vi "PWM In (subVI).vi"(0 "PWM Input":bool) -> (1 "Low Period":u32, 2 "High Period":u32)   [LabVIEW 2015]
doc: "This subVI supports a simple PWM measurement. An input signal is measured for its low period and high period."
panel:
  # "This subVI supports a simple PWM measurement.  An input signal is measured for its low period and high period."
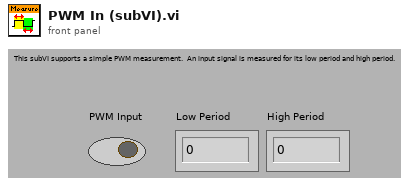
[diagram p1: front panel]
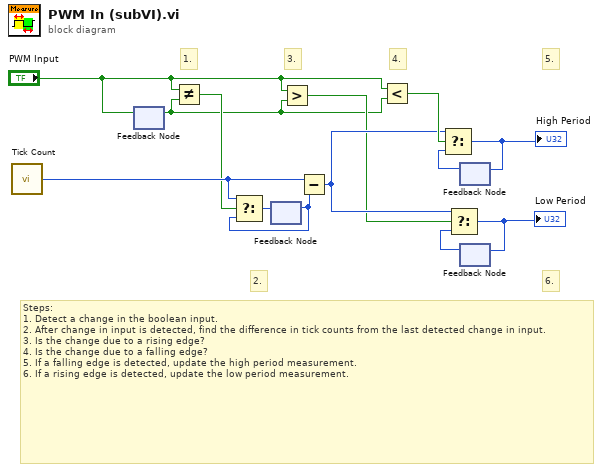
[diagram p0: block diagram]
diagram:
  # "Steps:\n1. Detect a change in the boolean input.\n2. After change in input is detected, find the difference in tick counts from the last detected change in input.\n3. Is the change due to a rising edge?\n4. Is the change due to a falling edge?\n5. If a falling edge is detected, update the high period measurement.\n6. If a rising edge is detected, update the low period measurement."
  # "5."
  # "6."
  # "2."
  # "4."
  # "3."
  # "1."
  n1 = call "Tick Count"() -> ("Tick Count(mSec)"=w13:u32)
  n2 = feedback-in #1("PWM Input") -> ()
  n3 = feedback #1() -> (w8:bool)  [unwired: 1 out]
  n4 = Not Equal?(x="PWM Input", y=w8) -> (x != y?=w9:bool)
  n5 = feedback #2() -> (w2:u32)  [unwired: 1 out]
  n6 = Select(t=w13, s=w9, f=w2) -> (s? t:f=w3:u32)
  n7 = feedback-in #2(w3) -> ()
  n8 = Greater?(x="PWM Input", y=w8) -> (0:w10:bool)
  n9 = Subtract(x=w13, y=w2) -> (x-y=w11:u32)
  n10 = Less?(x="PWM Input", y=w8) -> (x < y?=w12:bool)
  n11 = feedback #3() -> (w5:u32)  [unwired: 1 out]
  n12 = Select(t=w11, s=w12, f=w5) -> (s? t:f=w6:u32)
  "High Period" <- w6
  n13 = feedback-in #3(w6) -> ()
  n14 = feedback #4() -> (w4:u32)  [unwired: 1 out]
  n15 = Select(t=w11, s=w10, f=w4) -> (s? t:f=w7:u32)
  "Low Period" <- w7
  n16 = feedback-in #4(w7) -> ()
